vi "Get_ADAM_averages_client.vi"(6 "No of averages":i32=1, 7 "All Active Channels":bool, 9 "End time":dbl, 10 "Start time":dbl, 11 "ADAM Ch Names":string[](array[string])) -> (1 "Values":string[][](array[string]), 2 "Comments":string[](array[string]), 3 "Titles":string[](array[string]), 4 "Messages":string, 5 "DBL values":dbl[][](array[numeric]) format="%.2f")   [LabVIEW 2010]
doc: "This is an example of using features of the VI Server as a client. It shows how you might browse from one or more applications that may be exporting data from one or more data stations. \n\nThe example shows how to query a server for its list of exported VIs, how to get references to the VIs, and how call them with the Call By Reference function."
uses:
  Anemometry/Anemometry Sub Vis/Controls/Global_mode.ctl
  Sub VIs/ADAM Controls/Channel_names.ctl
  Anemometry/Anemometry Sub Vis/Globals/Preference_global.vi
panel:
  in  "vi type":refnum<vi>
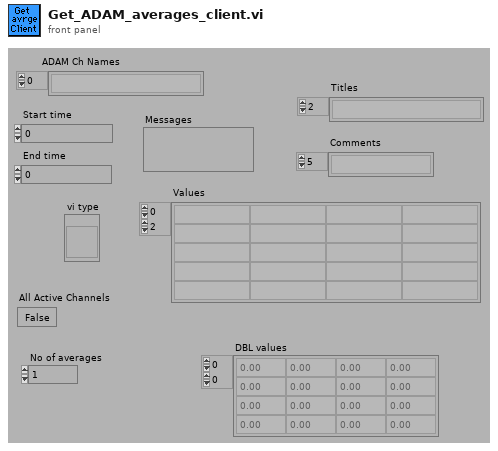
[diagram p1: front panel]
types:
  T1 = typedef "Global_mode.ctl" = enum16{"Read Global", "Load Global From File", "Write Global to File"}
  T2 = typedef "Channel_names.ctl" = enum16{"Active Only", "Active + Off", "All Channels"}
  T3 = typedef "Server_Comms.ctl" = enum16{"Server Link Healthy", "Do Not Link To Server"}
  T4 = typedef "Update_scan_value.ctl" = cluster{"Channel Name":string, "New Value":dbl}
  T5 = typedef "Ch_description_ADAM.ctl" = cluster{"Ch Name":string, "Type":T6, "Function":T7, "Ch State":T8, "Calibration type":T9, "A":dbl, "B":dbl, "C":dbl, "D":dbl, "Comments":string, "Address":T10, "String":string, "Duty":u16}
  T6 = typedef "Module_type_ADAM.ctl" = enum16{"4011", "4012", "4013", "4014", "4016", "4017", "4018", "4021", "4050", "4052", "4053", "4060", "4080", "5000", "5017", "5018", "5024", "5051", "5056", "5060", "6060", "Tracker", "WEST", "GILL", "JEM", "VICI", "Vaisala", "DRUCK", "Run VI Named:", "IR2100", "PPT", "Comparator", "VIRTUAL", "Hold Value", "Read A", "Read Ch", "Coded", "Client Info", "Web Client", "X10", "Test"}
  T7 = typedef "Function_ADAM.ctl" = enum16{"Analogue Input", "Digital Input", "Event counter", "Event rate", "Analogue Output", "Digital Output", "Relay Output"}
  T8 = typedef "Channel_State.ctl" = enum16{"On", "Off", "Always On", "Always Off"}
  T9 = typedef "Calib_type_ADAM.ctl" = enum16{"Raw", "Bx + A", "Cx^2 + Bx + A", "Dx^3 + Cx^2 + Bx + A", "In Band", "Hi-Tec Q", "Hi-Tec M_dot", "Text"}
  T10 = typedef "Address.ctl" = cluster{"Main":i32, "Ch.":i32, "Sub":i32, "Port Name":string}
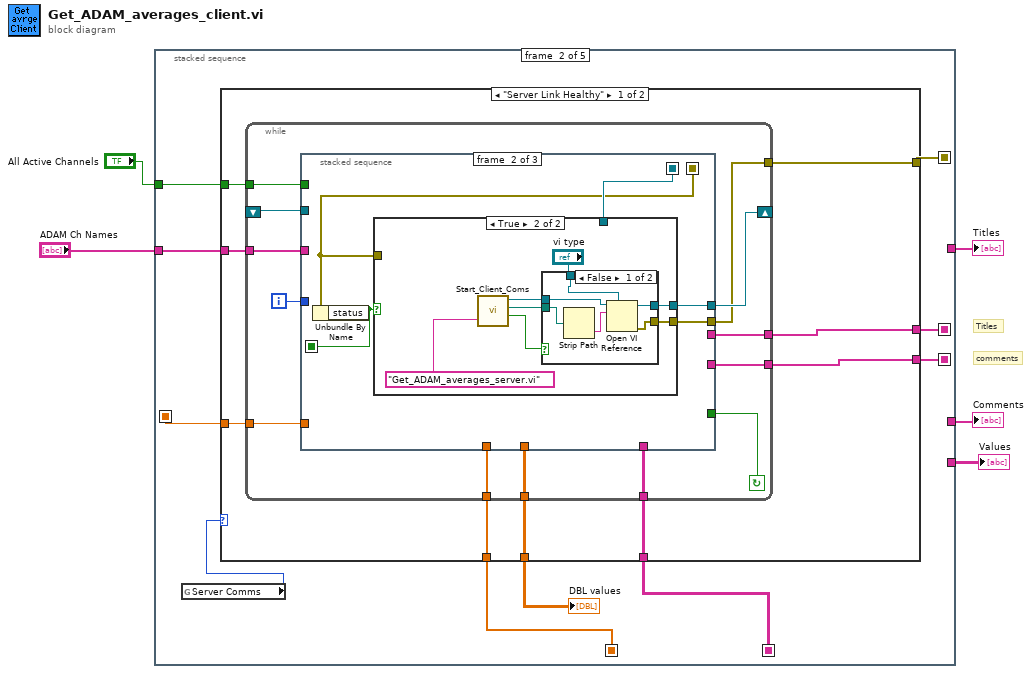
[diagram p0: block diagram]
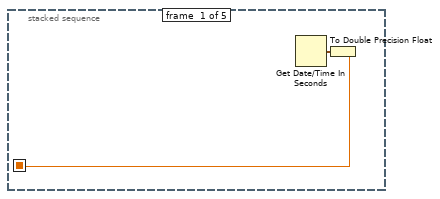
[diagram p2: hidden frame]
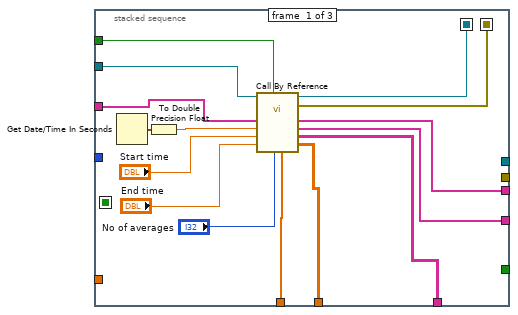
[diagram p3: hidden frame]
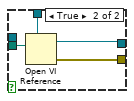
[diagram p5: hidden frame]
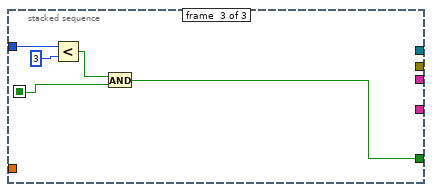
[diagram p6: hidden frame]
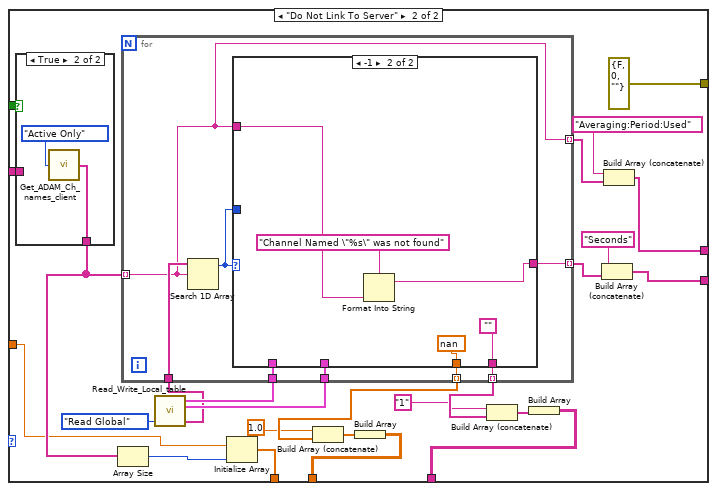
[diagram p7: hidden frame]
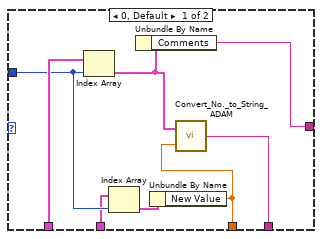
[diagram p9: hidden frame]
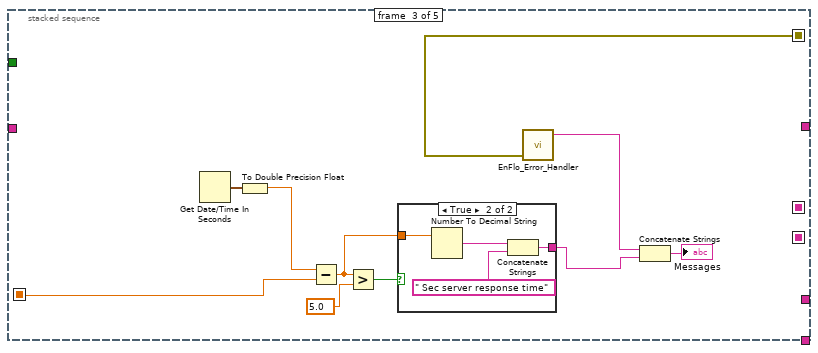
[diagram p10: hidden frame]
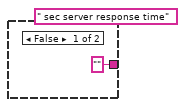
[diagram p11: hidden frame]
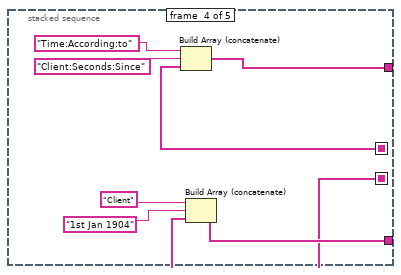
[diagram p12: hidden frame]
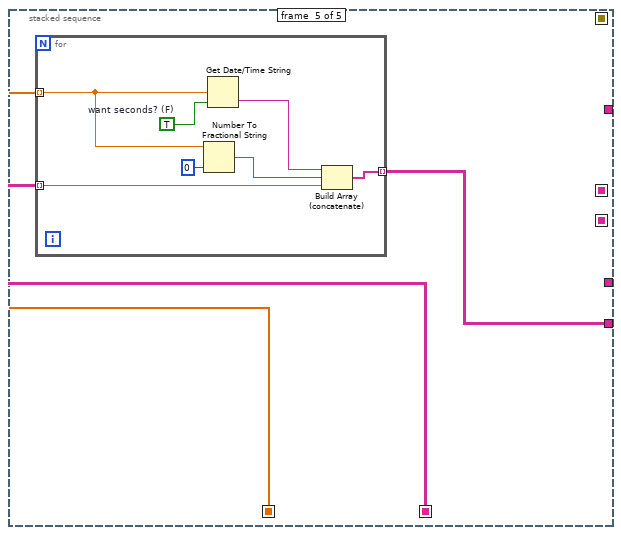
[diagram p13: hidden frame]
diagram:
  # "comments"
  # "Titles"
  n1 = stacked-sequence {
    seq-local: [_ w17 _ _ _] -> [_ _ _ w155 _]
    seq-local: [_ w8 _ _ _] -> [_ _ _ w148 _]
    seq-local: [_ w16 _ _ _] -> [_ _ _ _ w157]
    seq-local: [w7 _ _ _ _] -> [_ w15 w140 _ _]
    seq-local: [_ w14 _ _ _] -> [_ _ _ _ w158]
    seq-local: [_ w13 _ _ _] -> [_ _ w135 _ _]
    tunnel: [_ _ _ w153 _] -> w5
    tunnel: [_ _ _ w154 _] -> w4
    tunnel: [_ _ _ _ w156] -> w3
    tunnel: "ADAM Ch Names" -> [_ w10 _ _ _]
    tunnel: "All Active Channels" -> [_ w9 _ _ _]
    frame #0 {
      n2 = Get Date/Time In Seconds() -> (seconds since 1Jan1904=w6:timestamp)
      n3 = To Double Precision Float(number=w6) -> (double precision float=w7:dbl)
    }
    frame #1 {
      n4 = global read "Preference_global.vi" "Server Comms"() -> (w12:T3)
      n5 = case shown="\"Server Link Healthy\"" w12 {
        tunnel: [w26 w90] -> w17
        tunnel: [w25 w98] -> w16
        tunnel: w15 -> [w24 w88]
        tunnel: [w23 w104] -> w14
        tunnel: [w22 errorcluster {"status"=FALSE, "code"=0, "source"=""}] -> w13
        tunnel: [w21 w84] -> w11
        tunnel: w10 -> [w20 w99]
        tunnel: w9 -> [w19 w102]
        tunnel: [w18 w89] -> w8
        frame "Server Link Healthy" {
          n6 = while {
            tunnel: [w30] -> w22
            shift-left: _ -> [w34]
            shift-right: [w33] -> _
            tunnel: [w35] -> w23
            tunnel: w24 -> [w36]
            tunnel: [w37] -> w25
            tunnel: [w38] -> w18
            tunnel: [w39] -> w26
            tunnel: [w29] -> w21
            tunnel: w20 -> [w28]
            tunnel: w19 -> [w27]
            i -> [w32]
            stop <- w31 continue-if-true
            n7 = stacked-sequence {
              seq-local: [w44 _ _] -> [_ w58 _]
              seq-local: [w45 _ _] -> [_ w55 _]
              seq-local: [_ w57 _] -> [_ _ w80]
              tunnel: [w47 _ _] -> w39
              tunnel: [w52 _ _] -> w38
              tunnel: [w51 _ _] -> w37
              tunnel: w36 -> [_ _ _]
              tunnel: [w49 _ _] -> w35
              tunnel: w34 -> [w46 _ _]
              tunnel: [_ w59 _] -> w33
              tunnel: w32 -> [_ _ w81]
              tunnel: [_ _ w79] -> w31
              tunnel: [_ w56 _] -> w30
              tunnel: [w42 _ _] -> w29
              tunnel: w28 -> [w41 _ _]
              tunnel: w27 -> [w40 _ _]
              frame #0 {
                n8 = Get Date/Time In Seconds() -> (seconds since 1Jan1904=w43:timestamp)
                n9 = To Double Precision Float(number=w43) -> (double precision float=w53:dbl)
                n10 = call-by-ref "?"(reference=w46, "No of averages"="No of averages", "All Active Channels"=w40, "End time"="End time", "Start time"="Start time", "Clients time"=w53, "ADAM Ch Names"=w41) -> (reference out=w44:refnum<vi>, error out=w45:errorcluster, "DBL values"=w42:dbl[][], "Values"=w51:string[][], "Comments"=w52:string[], "Titles"=w47:string[], "Times"=w49:dbl[])  [unwired: 1 in]
              }
              frame #1 {
                n11 = Unbundle By Name(w55) -> ("status"=w57:bool)
                n12 = case shown="True" w57 {
                  tunnel: [w61 w64] -> w59
                  tunnel: w58 -> [w61 _]
                  tunnel: [w60 w62] -> w56
                  tunnel: w55 -> [w60 _]
                  frame False {
                  }
                  frame True {
                    n13 = call "Start_Client_Coms.vi"("VI name to run on server"="Get_ADAM_averages_server.vi") -> ("LabVIEW application reference"=w66:refnum<vi>, "Checked VI name"=w67:path, "Local Call"=w65:bool)  [unwired: 1 in, 1 out]
                    n14 = case shown="False" w65 {
                      tunnel: [w72 w78] -> w64
                      tunnel: "vi type" -> [w71 w77]
                      tunnel: w67 -> [w70 w76]
                      tunnel: w66 -> [w69 _]
                      tunnel: [w73 w75] -> w62
                      frame False {
                        n15 = Strip Path(path=w70) -> (name=w74:string)  [unwired: 1 out]
                        n16 = Open VI Reference(type specifier VI Refnum (for type only)=w71, application reference (local)=w69, vi path=w74) -> (vi reference=w72:refnum<vi>, error out=w73:errorcluster)  [unwired: 1 in, 2 out]
                      }
                      frame True {
                        n17 = Open VI Reference(type specifier VI Refnum (for type only)=w77, vi path=w76) -> (vi reference=w78:refnum<vi>, error out=w75:errorcluster)  [unwired: 1 in, 3 out]
                      }
                    }
                  }
                }
              }
              frame #2 {
                n18 = Less?(x=w81, y=3) -> (x < y?=w82:bool)
                n19 = And(x=w82, y=w80) -> (x .and. y?=w79:bool)
              }
            }
          }
        }
        frame "Do Not Link To Server" {
          n20 = case shown="True" w102 {
            tunnel: [w109 w110] -> w101
            tunnel: w99 -> [w109 _]
            frame False {
            }
            frame True {
              n21 = call "Get_ADAM_Ch_names_client.vi"("Channel names set"=Channel_names."Active Only") -> ("Ch names"=w110:string[])
            }
          }
          n22 = Array Size(array=w101) -> (size(s)=w105:i32)
          n23 = call "Read_Write_Local_table.vi"("Mode"=Global_mode."Read Global") -> ("Ch Names"=w100:string[], "Ch Values Out"=w106:T4[], "Channels Descriptions Out"=w107:T5[])  [unwired: 2 in]
          n24 = for {
            tunnel: w100 -> [w116]
            tunnel: w101 -> [w115] mode=indexing
            tunnel: w107 -> [w118]
            tunnel: w106 -> [w117]
            tunnel: [w115] -> w91 mode=indexing
            tunnel: [w114] -> w95 mode=indexing
            tunnel: [w113] -> w97 mode=indexing
            tunnel: [w112] -> w87 mode=indexing
            n25 = Search 1D Array(1D array=w116, element=w115) -> (index of element=w119:i32)  [unwired: 1 out]
            n26 = case shown="-1" w119 {
              tunnel: w119 -> [w126 _]
              tunnel: w118 -> [w127 _]
              tunnel: w117 -> [w125 _]
              tunnel: w115 -> [_ w132]
              tunnel: [w122 w130] -> w114
              tunnel: [w121 ""] -> w113
              tunnel: [w120 nan ("New Value")] -> w112
              frame 0, Default {
                n27 = Index Array(array=w127, index=w126) -> (element=w123:T5)
                n28 = Index Array(array=w125, index=w126) -> (element=w124:T4)
                n29 = Unbundle By Name(w123) -> ("Comments"=w122:string)
                n30 = Unbundle By Name(w124) -> ("New Value"=w120:dbl)
                n31 = call "Convert_No._to_String_ADAM.vi"("Input number"=w120, "Ch Description"=w123) -> ("Output sting"=w121:string)
              }
              frame -1 {
                n32 = Format Into String(format string="Channel Named \"%s\" was not found" ("Format String"), w132) -> (resulting string=w130:string)  [unwired: 2 in, 1 out]
              }
            }
          }
          n33 = Initialize Array(w88, w105) -> (w104:dbl[])
          n34 = Build Array (concatenate)(1.0, w87) -> (w85:dbl[])
          n35 = Build Array(w85) -> (w84:dbl[][])
          n36 = Build Array (concatenate)("1", w97) -> (w96:string[])
          n37 = Build Array(w96) -> (w98:string[][])
          n38 = Build Array (concatenate)("Seconds", w95) -> (w89:string[])
          n39 = Build Array (concatenate)("Averaging:Period:Used", w91) -> (w90:string[])
        }
      }
      "DBL values" <- w11
    }
    frame #2 {
      n40 = Get Date/Time In Seconds() -> (seconds since 1Jan1904=w133:timestamp)
      n41 = To Double Precision Float(number=w133) -> (double precision float=w141:dbl)
      n42 = Subtract(x=w141, y=w140) -> (x-y=w137:dbl)
      n43 = Greater?(x=w137, y=5.0) -> (0:w138:bool)
      n44 = case shown="True" w138 {
        tunnel: w137 -> [_ w147]
        tunnel: ["" w144] -> w136
        frame False {
          (unwired) " sec server response time"
        }
        frame True {
          n45 = Number To Decimal String(number=w147) -> (decimal integer string=w145:string)  [unwired: 1 out]
          n46 = Concatenate Strings(w145, " Sec server response time") -> (w144:string)
        }
      }
      n47 = call "EnFlo_Error_Handler.vi"("error in (no error)"=w135) -> ("Email Message"=w134:string)  [unwired: 2 in, 2 out]
      n48 = Concatenate Strings(w134, w136) -> (→"Messages":string)
    }
    frame #3 {
      n49 = Build Array (concatenate)("Time:According:to", "Client:Seconds:Since", w155) -> (w153:string[])
      n50 = Build Array (concatenate)("Client" ("Comments"), "1st Jan 1904" ("Comments"), w148) -> (w154:string[])
    }
    frame #4 {
      n51 = for {
        tunnel: w158 -> [w160] mode=indexing
        tunnel: [w165] -> w156 mode=indexing
        tunnel: w157 -> [w164] mode=indexing
        w163 = TRUE  # want seconds? (F)
        n52 = Number To Fractional String(number=w160, precision (6)=i16 0) -> (F-format string=w159:string)  [unwired: 2 out]
        n53 = Get Date/Time String(seconds (now)=w160, want seconds? (F)=w163) -> (time string=w162:string)  [unwired: 2 out]
        n54 = Build Array (concatenate)(w162, w159, w164) -> (w165:string[])
      }
    }
  }
  "Titles" <- w5
  "Comments" <- w4
  "Values" <- w3
